vi "修改Email服务器配置.vi"(11 "邮件服务器配置":T1) -> (0 "error out":errorcluster caption="错误输出")   [LabVIEW 2013, in "Admin客户端.lvclass"]
uses:
  <vilib>/Utility/config.llb/Write Key (String).vi
  <vilib>/Utility/config.llb/NI_LVConfig.lvlib
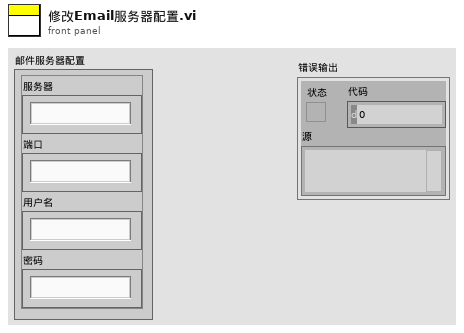
[diagram p1: front panel]
types:
  T1 = cluster{"服务器":string, "端口":string, "用户名":string, "密码":string}
  T2 = typedef "NI_LVConfig.lvlib/Config Data RefNum.ctl" = refnum<k1>
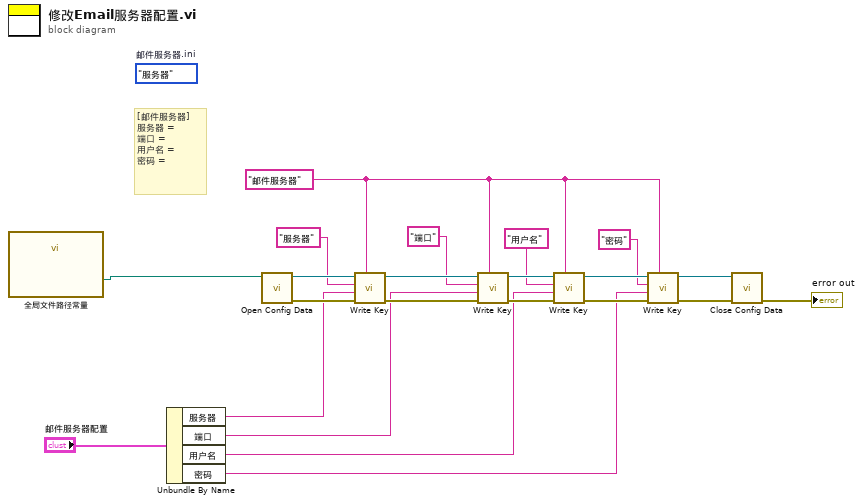
[diagram p0: block diagram]
diagram:
  w13 = "邮件服务器" ("section")
  (unwired) enum16{"服务器", "端口", "用户名", "密码"}."服务器"  # 邮件服务器.ini
  # "[邮件服务器]\n服务器 =\n端口 =\n用户名 =\n密码 ="
  n1 = call "全局文件路径常量.vi"() -> ("Email服务器配置"=w22:path)  [unwired: 9 in, 2 out]
  n2 = Unbundle By Name("邮件服务器配置") -> ("服务器"=w5:string, "端口"=w4:string, "用户名"=w3:string, "密码"=w2:string)
  n3 = call <vilib>:"Open Config Data.vi"("configuration file path"=w22) -> ("error out"=w17:errorcluster, "refnum"=w21:T2)  [unwired: 8 in, 1 out]
  n4 = call-poly <vilib>:"Write Key.vi"("section"=w13, "error in (no error)"=w17, "value"=w5, "key"="服务器" ("section"), "refnum"=w21) -> ("error out"=w16:errorcluster, "refnum out"=w20:T2)  [unwired: 4 in, 1 out]
  n5 = call-poly <vilib>:"Write Key.vi"("section"=w13, "error in (no error)"=w16, "value"=w4, "key"="端口" ("section"), "refnum"=w20) -> ("error out"=w15:errorcluster, "refnum out"=w19:T2)  [unwired: 4 in, 1 out]
  n6 = call-poly <vilib>:"Write Key.vi"("section"=w13, "error in (no error)"=w15, "value"=w3, "key"="用户名" ("section"), "refnum"=w19) -> ("error out"=w14:errorcluster, "refnum out"=w18:T2)  [unwired: 4 in, 1 out]
  n7 = call-poly <vilib>:"Write Key.vi"("section"=w13, "error in (no error)"=w14, "value"=w2, "key"="密码" ("section"), "refnum"=w18) -> ("error out"=w11:errorcluster, "refnum out"=w12:T2)  [unwired: 4 in, 1 out]
  n8 = call <vilib>:"Close Config Data.vi"("error in (no error)"=w11, "refnum"=w12) -> ("error out"=→"error out":errorcluster)  [unwired: 8 in, 1 out]
